vi "Write Both Fan States.vi"(8 "error in (no error)":errorcluster, 9 "Fan B State":bool, 10 "Fan A State":bool, 11 "Simulated Dual Fan in":refnum<class "Simulated Dual Fan.lvclass">) -> (0 "error out":errorcluster)   [LabVIEW 2018, in "Simulated Dual Fan.lvclass"]
uses:
  Simulated Dual Fan.lvclass
  Cooler Plug-Ins/Simulated Evaporative Cooler.lvclass/Simulation Data_Global.vi
  Cooler Plug-Ins/Simulated Evaporative Cooler.lvclass/Simulated Evaporative Cooler.lvclass
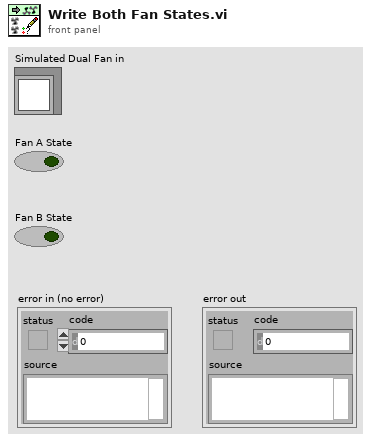
[diagram p1: front panel]
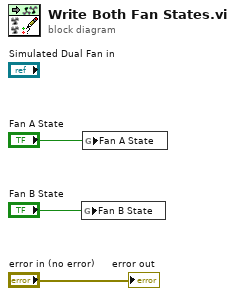
[diagram p0: block diagram]
diagram:
  n1 = global write "Simulation Data_Global.vi" "Fan B State"("Fan B State") -> ()
  n2 = global write "Simulation Data_Global.vi" "Fan A State"("Fan A State") -> ()
  "error out" <- "error in (no error)"
